vi "GetStabilityData.vi"(0 "ProvidedData":dbl[](array[numeric]), 5 "MinIndex":dbl, 7 "MaxIndex":dbl, 9 "MeanIndex":dbl, 11 "StdDevIndex":dbl) -> (10 "ReturnData":dbl[](array[numeric]))   [LabVIEW 2016]
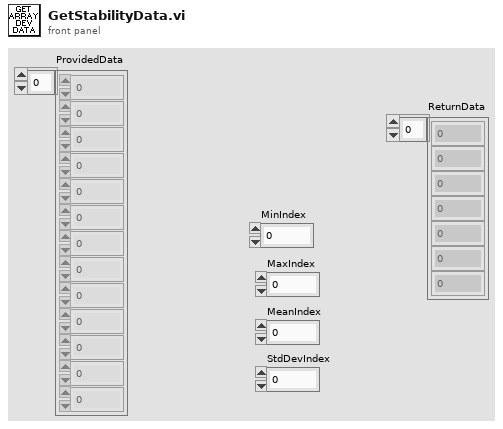
[diagram p1: front panel]
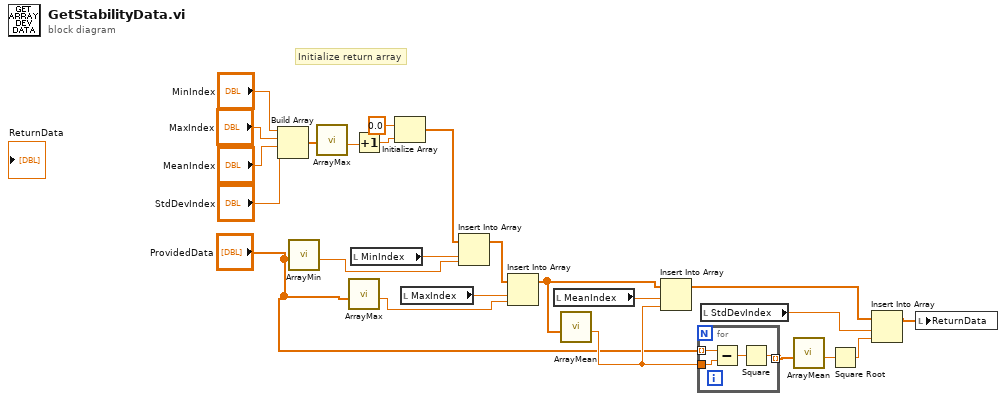
[diagram p0: block diagram]
diagram:
  # "Initialize return array"
  n1 = Build Array("MinIndex", "MaxIndex", "MeanIndex", "StdDevIndex") -> (w19:dbl[])
  n2 = call "ArrayMin.vi"("Array"="ProvidedData") -> ("min"=w16:dbl)  [unwired: 10 in]
  n3 = call "ArrayMax.vi"("Array"=w19) -> ("max"=w18:dbl)  [unwired: 10 in]
  n4 = call "ArrayMax.vi"("Array"="ProvidedData") -> ("max"=w2:dbl)  [unwired: 10 in]
  n5 = local read "MinIndex"() -> (w15:dbl)
  n6 = Increment(x=w18) -> (x+1=w17:dbl)
  n7 = Initialize Array(0.0 ("element"), w17) -> (w7:dbl[])
  n8 = local read "MaxIndex"() -> (w14:dbl)
  n9 = Insert Into Array(array=w7, index=w15, new element=w16) -> (w6:dbl[])
  n10 = Insert Into Array(array=w6, index=w14, new element=w2) -> (w5:dbl[])
  n11 = local read "MeanIndex"() -> (w8:dbl)
  n12 = call "ArrayMean.vi"("Array"=w5) -> ("Mean"=w4:dbl)  [unwired: 10 in]
  n13 = Insert Into Array(array=w5, index=w8, new element=w4) -> (w3:dbl[])
  n14 = for {
    tunnel: [w27] -> w12 mode=indexing
    tunnel: w4 -> [w26]
    tunnel: "ProvidedData" -> [w25] mode=indexing
    n15 = Subtract(x=w25, y=w26) -> (x-y=w28:dbl)
    n16 = Square(x=w28) -> (x^2=w27:dbl)
  }
  n17 = local read "StdDevIndex"() -> (w9:dbl)
  n18 = call "ArrayMean.vi"("Array"=w12) -> ("Mean"=w13:dbl)  [unwired: 10 in]
  n19 = Square Root(x=w13) -> (sqrt(x)=w11:dbl)
  n20 = Insert Into Array(array=w3, index=w9, new element=w11) -> (w10:dbl[])
  n21 = local write "ReturnData"(w10) -> ()
